vi "Compute DistanceToTarget2.vi"(7 "Boiler?":bool=TRUE, 8 "Calibrated":bool, 9 "Camera Type":T6, 10 "Line":T4, 11 "Image Src":T5) -> (1 "Edges":cluster{"X":sgl, "Y":sgl}[](array[cluster]), 2 "Distance (ft)":dbl, 3 "Image Dst Out":T5)   [LabVIEW 2016]
doc: "Using the camera lens information and the real world size of the target, use trig and ratios to determine the distance to the target. Also returns the location relative to the image center in a (-1 , 1) coordinate system that may be useful for steering the robot."
uses:
  Camera Types.ctl
  <vilib>/vision/Image Controls.llb/IMAQ Image.ctl
  <vilib>/vision/Measure.llb/Edge New.ctl
  <vilib>/vision/Measure.llb/Edge Options.ctl
  <vilib>/vision/Measure.llb/Edge Polarity.ctl
  <vilib>/vision/NI_Vision_Development_Module.lvlib
panel:
  in  "Edge Options":T1={"Edge Polarity"=0, "Kernel Size"=3, "Width"=3, "Minimum Edge Strength"=30.0, "Interpolation Type"=enum."Bilinear Fixed", "Data Processing Method"=enum."Average"} {"Edge Polarity" items=["All Edges", "Rising Edges", "Falling Edges"]; "Minimum Edge Strength" format="%.2f"; "Width" step=2; "Kernel Size" step=2}
  out "lengths":dbl[](array[numeric])
  out "Edge Information":T3[](array[typedef]) {"Distance (Real-World)" format="%.2f"; "Location (Real-World)"."Y" format="%.2g"; "Location (Real-World)"."X" format="%.2f"; "Noise" format="%.2f"; "Location (Pixel)"."Y" format="%.2g"; "Location (Pixel)"."X" format="%.2f"; "Strength" format="%.2f"; "Distance (Pixel)" format="%.2f"}
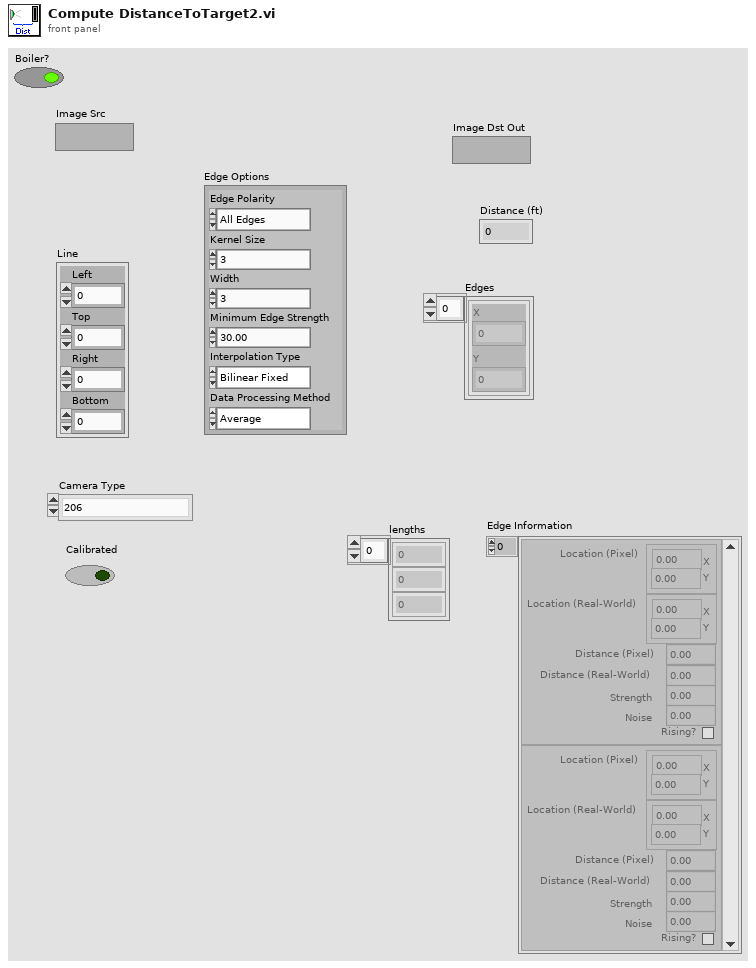
[diagram p1: front panel]
types:
  T1 = typedef "Edge Options.ctl" = cluster{"Edge Polarity":T2, "Kernel Size":u32, "Width":u32, "Minimum Edge Strength":sgl, "Interpolation Type":enum32{"Zero Order", "Bilinear", "Quadratic", "Cubic", "Bilinear Fixed"}, "Data Processing Method":enum32{"Average", "Median"}}
  T2 = typedef "Edge Polarity.ctl" = u32
  T3 = typedef "Edge New.ctl" = cluster{"Location (Pixel)":cluster{"X":sgl, "Y":sgl}, "Location (Real-World)":cluster{"X":sgl, "Y":sgl}, "Distance (Pixel)":dbl, "Distance (Real-World)":dbl, "Strength":dbl, "Noise":dbl, "Rising?":bool}
  T4 = cluster{"Left":dbl, "Top":dbl, "Right":dbl, "Bottom":dbl}
  T5 = typedef "IMAQ Image.ctl" = refnum<image>
  T6 = typedef "Camera Types.ctl" = enum16{"206", "1011", "1013", "MS HD3000 square", "MS HD3000 640x480"}
  T7 = enum16{"Get First Edge", "Get First + Last Edge", "Get All Edges", "Get Best Edge"}
  T8 = typedef "ROI Descriptor" = cluster{"Global Rectangle":i32[], "Contours":cluster{"ID":enum32{"External", "Internal"}, "Type":u32, "Coordinates":i32[]}[]}
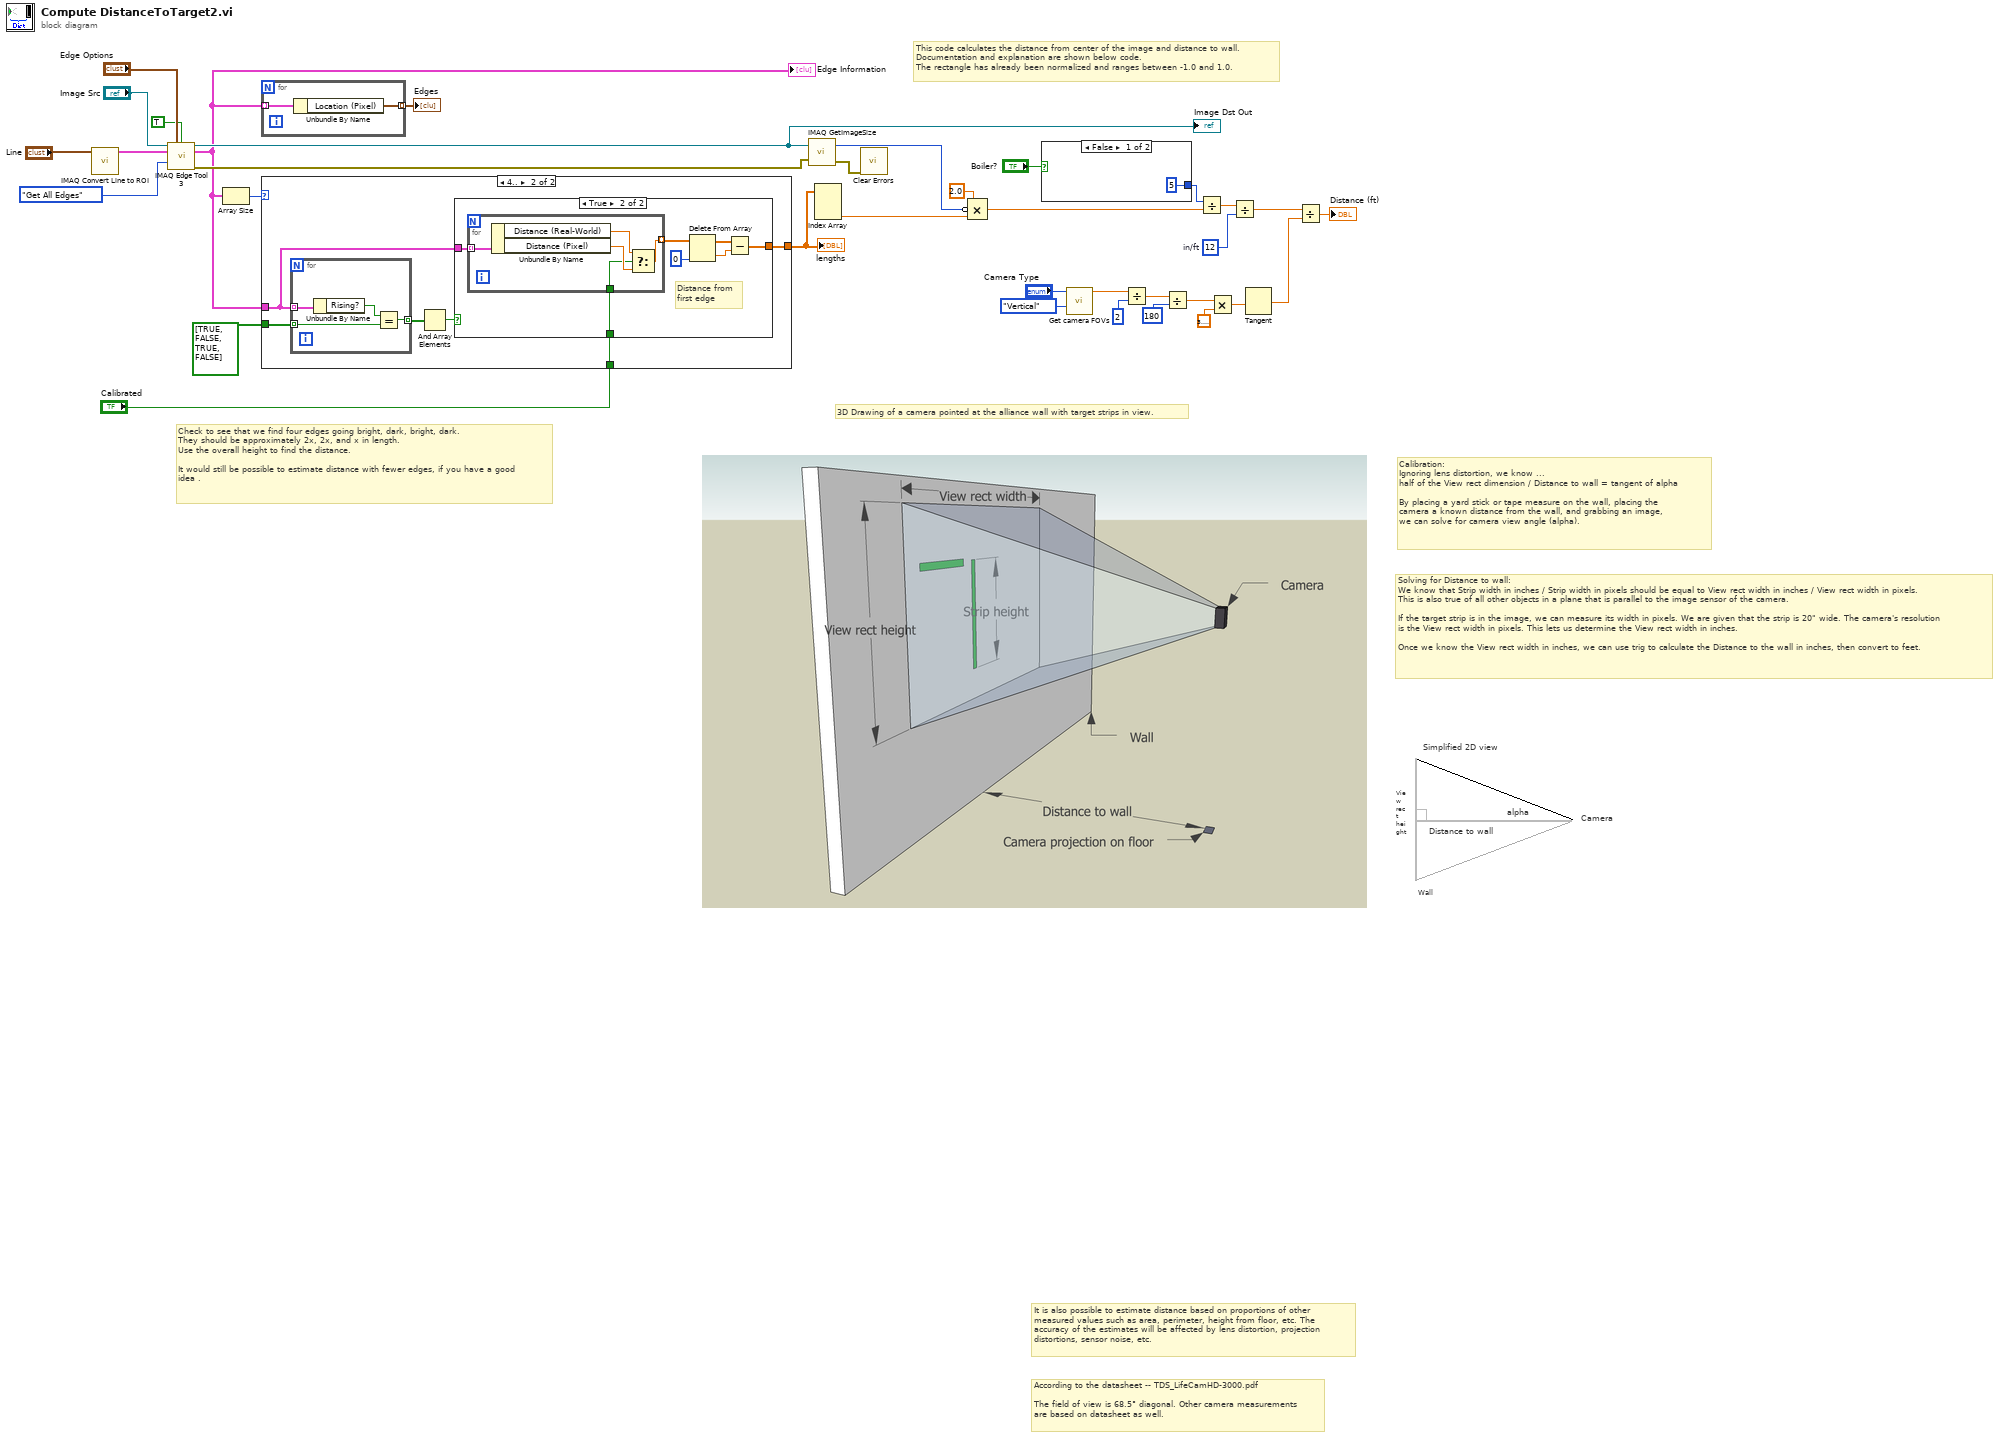
[diagram p0: block diagram]
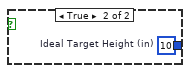
[diagram p2: hidden frame]
diagram:
  w29 = 12  # in/ft
  # "Check to see that we find four edges going bright, dark, bright, dark.\nThey should be approximately 2x, 2x, and x in length.\nUse the overall height to find the distance.\n\nIt would still be possible to estimate distance with fewer edges, if you have a good\nidea ."
  # "It is also possible to estimate distance based on proportions of other\nmeasured values such as area, perimeter, height from floor, etc. The\naccuracy of the estimates will be affected by lens distortion, projection\ndistortions, sensor noise, etc."
  # "According to the datasheet -- TDS_LifeCamHD-3000.pdf\n\nThe field of view is 68.5° diagonal. Other camera measurements\nare based on datasheet as well."
  # "Wall"
  # "Camera"
  # "Simplified 2D view"
  # "Solving for Distance to wall:\nWe know that Strip width in inches / Strip width in pixels should be equal to View rect width in inches / View rect width in pixels.\nThis is also true of all other objects in a plane that is parallel to the image sensor of the camera.\n\nIf the target strip is in the image, we can measure its width in pixels. We are given that the strip is 20\" wide. The camera's resolution\nis the View rect width in pixels. This lets us determine the View rect width in inches.\n\nOnce we know the View rect width in inches, we can use trig to calculate the Distance to the wall in inches, then convert to feet."
  # "3D Drawing of a camera pointed at the alliance wall with target strips in view."
  # "Distance to wall"
  # "View rect height"
  # "alpha"
  # "Calibration:\nIgnoring lens distortion, we know ...\nhalf of the View rect dimension / Distance to wall = tangent of alpha\n\nBy placing a yard stick or tape measure on the wall, placing the\ncamera a known distance from the wall, and grabbing an image,\nwe can solve for camera view angle (alpha)."
  # "This code calculates the distance from center of the image and distance to wall.\nDocumentation and explanation are shown below code.\nThe rectangle has already been normalized and ranges between -1.0 and 1.0."
  n1 = call "IMAQ Convert Line to ROI"("Line"="Line") -> ("ROI Descriptor"=w19:T8)  [unwired: 8 in, 1 out]
  n2 = call "IMAQ Edge Tool 3"("Image"="Image Src", "Edge Options"="Edge Options", "Optimized Mode"=TRUE, "ROI Descriptor"=w19, "Process"=T7."Get All Edges") -> ("Image (duplicate)"=w4:T5, "Edge Information"=w3:T3[], "error out"=w8:errorcluster)  [unwired: 6 in, 2 out]
  "Image Dst Out" <- w4
  "Edge Information" <- w3
  n3 = Array Size(array=w3) -> (size(s)=w15:i32)
  n4 = for {
    tunnel: w3 -> [w37] mode=indexing
    tunnel: [w36] -> w2 mode=indexing
    n5 = Unbundle By Name(w37) -> ("Location (Pixel)"=w36:cluster{"X":sgl, "Y":sgl})
  }
  "Edges" <- w2
  n6 = case shown="4.." w15 {
    tunnel: w3 -> [_ w40]
    tunnel: bool[] [TRUE, FALSE, TRUE, FALSE] -> [_ w43]
    tunnel: [_ w39] -> w13
    tunnel: "Calibrated" -> [_ w38]
    frame 0, Default {
    }
    frame 4.. {
      n7 = for {
        tunnel: w40 -> [w59] mode=indexing
        tunnel: w43 -> [w57] mode=indexing
        tunnel: [w56] -> w42 mode=indexing
        n8 = Unbundle By Name(w59) -> ("Rising?"=w58:bool)
        n9 = Equal?(x=w58, y=w57) -> (x = y?=w56:bool)
      }
      n10 = And Array Elements(Boolean array=w42) -> (logical AND=w41:bool)
      n11 = case shown="True" w41 {
        tunnel: w40 -> [_ w50]
        tunnel: [_ w46] -> w39
        tunnel: w38 -> [_ w44]
        frame False {
        }
        frame True {
          # "Distance from\nfirst edge"
          n12 = for {
            tunnel: w50 -> [w55] mode=indexing
            tunnel: [w53] -> w49 mode=indexing
            tunnel: w44 -> [w51]
            n13 = Unbundle By Name(w55) -> ("Distance (Real-World)"=w54:dbl, "Distance (Pixel)"=w52:dbl)
            n14 = Select(t=w54, s=w51, f=w52) -> (s? t:f=w53:dbl)
          }
          n15 = Delete From Array(array=w49, index=0) -> (deleted portion=w45:dbl, array with subset deleted=w47:dbl[])  [unwired: 1 in]
          n16 = Subtract(x=w47, y=w45) -> (x-y=w46:dbl[])
        }
      }
    }
  }
  "lengths" <- w13
  n17 = call "IMAQ GetImageSize"("Image"=w4, "error in (no error)"=w8) -> ("Y Resolution"=w9:i32, "error out"=w7:errorcluster)  [unwired: 2 in, 1 out]
  n18 = Index Array(array=w13) -> (element #3=w11:dbl)  [unwired: 3 in, 2 out]
  n19 = call <vilib>:"Clear Errors.vi"("error in (no error)"=w7) -> ()  [unwired: 5 in, 2 out]
  n20 = Compound Arithmetic op=MULTIPLY(2.0, invert w9, w11) -> (w10:dbl)
  n21 = case shown="False" "Boiler?" {
    tunnel: [5 ("Ideal Target Height (in)") w61] -> w22
    frame False {
    }
    frame True {
      w61 = 10  # Ideal Target Height (in)
    }
  }
  n22 = call "Get camera FOVs.vi"("Type"=enum16{"Horizontal", "Vertical", "Diagonal"}."Vertical" ("Angle"), "Camera Type"="Camera Type") -> ("FOV"=w24:dbl)  [unwired: 8 in, 1 out]
  n23 = Divide(x=w24, y=2) -> (x/y=w32:dbl)
  n24 = Divide(x=w32, y=180) -> (x/y=w31:dbl)
  n25 = Divide(x=w22, y=w10) -> (x/y=w26:dbl)
  n26 = Multiply(x=w31, y=3.141592653589793) -> (x*y=w33:dbl)
  n27 = Divide(x=w26, y=w29) -> (x/y=w25:dbl)
  n28 = Tangent(1:w33) -> (0:w28:dbl)
  n29 = Divide(x=w25, y=w28) -> (x/y=→"Distance (ft)":dbl)
